vi "log_z.vi"(8 "error in (no error)":errorcluster, 9 "focus value":sgl, 10 "ZPos":dbl, 11 "log file in":refnum<file>) -> (0 "error out":errorcluster, 3 "log file out":refnum<file>)   [LabVIEW 2011]
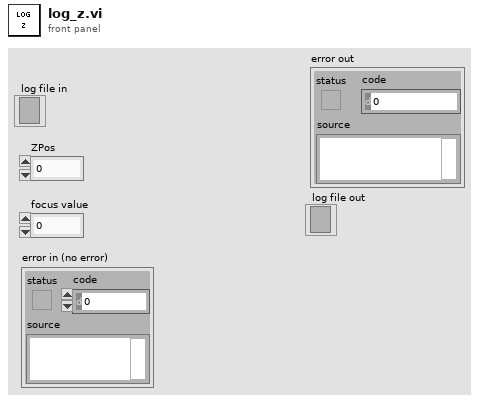
[diagram p1: front panel]
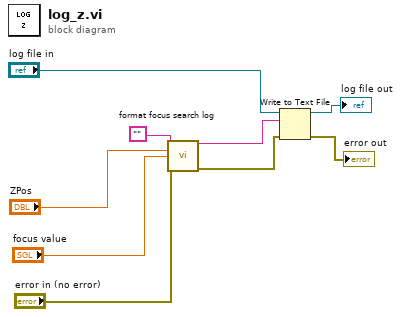
[diagram p0: block diagram]
diagram:
  n1 = call "format focus search log"("Beginning Text"="", "Z"="ZPos", "focus value"="focus value", "error in (no error)"="error in (no error)") -> ("Result"=w7:string, "error out"=w8:errorcluster)  [unwired: 10 in]
  n2 = Write to Text File(file (use dialog)="log file in", text=w7, error in=w8) -> (refnum out=→"log file out":refnum<file>, error out=→"error out":errorcluster)  [unwired: 1 in, 1 out]
